vi "Init Trigger.vi"(8 "error in (no error)":errorcluster, 11 "Trigger in":T1 {"Node Data Ref" format="%.0x"; "Node ID" format="%.0x"}) -> (0 "error out":errorcluster, 3 "Trigger out":T1 {"Node Data Ref" format="%.0x"; "Node ID" format="%.0x"})   [LabVIEW 2015, in "Waveform Data Logger Engine.lvlib"]
uses:
  Waveform Data Logger Engine.lvlib
  Types/Trigger Settings.ctl
  Classes/Triggers/Trigger/Trigger.lvclass
  <vilib>/NI Veristand/Custom Device API/Custom Device Item Ref.ctl
  Classes/Triggers/Trigger/Trigger.lvclass/Trigger.ctl
  Classes/Triggers/Digital Edge Trigger/Digital Edge Trigger.lvclass/Digital Edge Trigger.ctl
  Classes/Triggers/Analog Edge Trigger/Analog Edge Trigger.lvclass/Analog Edge Trigger.ctl
  Classes/Triggers/Value Change Trigger/Value Change Trigger.lvclass/Value Change Trigger.ctl
  Classes/Triggers/Digital Edge Trigger/Initialize Digital Edge Trigger.vi
  Classes/Triggers/Analog Edge Trigger/Initialize Analog Edge Trigger.vi
  Classes/Triggers/Value Change Trigger/Initialize Value Change Trigger.vi
  Classes/Triggers/Value Change Trigger/Value Change Trigger.lvclass
  Classes/Triggers/Analog Edge Trigger/Analog Edge Trigger.lvclass
  Classes/Triggers/Digital Edge Trigger/Digital Edge Trigger.lvclass
  <vilib>/NI VeriStand/Custom Device API/Custom Device API.lvlib
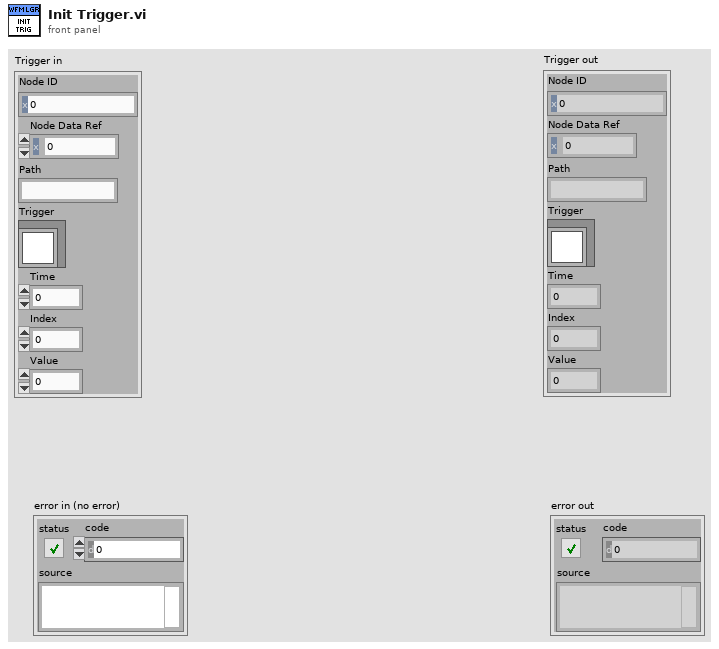
[diagram p1: front panel]
types:
  T1 = typedef "Waveform Data Logger Engine.lvlib/Trigger Settings.ctl" = cluster{"Node ID":T2, "Node Data Ref":i32, "Path":string, "Trigger":refnum<class "Trigger.lvclass">, "Time":dbl, "Index":i32, "Value":dbl}
  T2 = typedef "Custom Device API.lvlib/Custom Device Item Ref.ctl" = u64
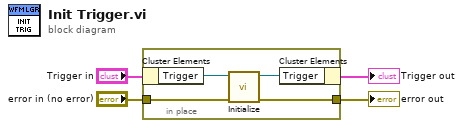
[diagram p0: block diagram]
diagram:
  n1 = in-place {
    in-place-border: "error in (no error)" -> [w8]
    in-place-border: [w7] -> w3
    n2 = in-place-cluster #1("Trigger in") -> ("Trigger"=w6:refnum<class "Trigger.lvclass">)
    n3 = call "Initialize.vi"("error in (no error)"=w8, "Trigger in"=w6) -> ("error out"=w7:errorcluster, "Trigger out"=w5:refnum<class "Trigger.lvclass">)  [unwired: 8 in]
    n4 = in-place-cluster #1("Trigger"=w5) -> (→"Trigger out":T1)
  }
  "error out" <- w3
